vi "Model Recognition.vi"(8 "error in (no error)":errorcluster, 10 "Model Type (0: N5181A)":u16(ring) items=["N5181A"=0, "N5182A"=1, "N5183A"=2, "E8241A"=5, "E8244A"=6, "E8251A"=7, "E8254A"=8, "E8247C"=10, "E8257C"=11, "E8267C"=12, "E8257D"=15, "E8267D"=16], 11 "VISA resource name":refnum<visa-resource-name>) -> (0 "error out":errorcluster, 2 "Is Model Correct":bool, 3 "VISA resource name out":refnum<visa-resource-name>)   [LabVIEW 2012, in "Agilent PSG MXG Series.lvlib"]
doc: "Specifies whether the model type is correct."
uses:
  Agilent PSG MXG Series.lvlib
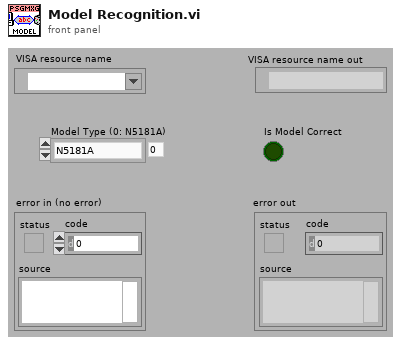
[diagram p1: front panel]
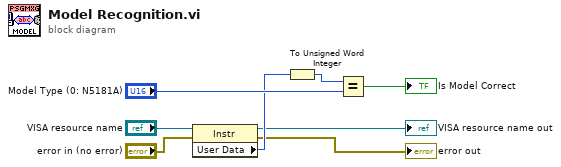
[diagram p0: block diagram]
diagram:
  n1 = property class="Instr"(reference="VISA resource name", error in="error in (no error)") -> (reference out=→"VISA resource name out":refnum<visa-resource-name>, error out=→"error out":errorcluster, "User Data"=w3:u32)
  n2 = To Unsigned Word Integer(number=w3) -> (unsigned 16bit integer=w8:u16)
  n3 = Equal?(x=w8, y="Model Type (0: N5181A)") -> (x = y?=→"Is Model Correct":bool)
